vi "Bulk Delete Prompt.vi"(8 "error in (no error)":errorcluster, 11 "Item Ref in":T1 format="%.0x") -> (0 "error out":errorcluster)   [LabVIEW 2015, in "Modbus Master System Explorer.lvlib"]
uses:
  Modbus Master System Explorer.lvlib
  <vilib>/NI Veristand/Custom Device API/Custom Device Item Ref.ctl
  <vilib>/NI VeriStand/Custom Device API/Custom Device API.lvlib
panel:
  in  "Cancel":bool
  in  "Delete Selected":bool
  in  "Channels":i32[](listbox)
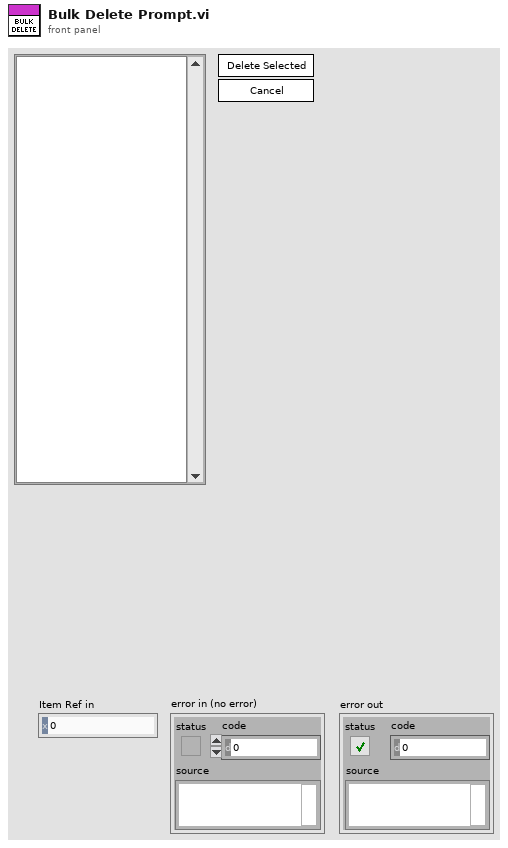
[diagram p1: front panel]
types:
  T1 = typedef "Custom Device API.lvlib/Custom Device Item Ref.ctl" = u64
  T2 = enum32{"Invalid", "Standard", "Closed", "Hidden", "Minimized", "Maximized"}
  T3 = typedef "Custom Device API.lvlib/Custom Device Item Info.ctl" = cluster{"Name":string, "Is Channel":bool, "GUID":string, "Is Waveform":bool}
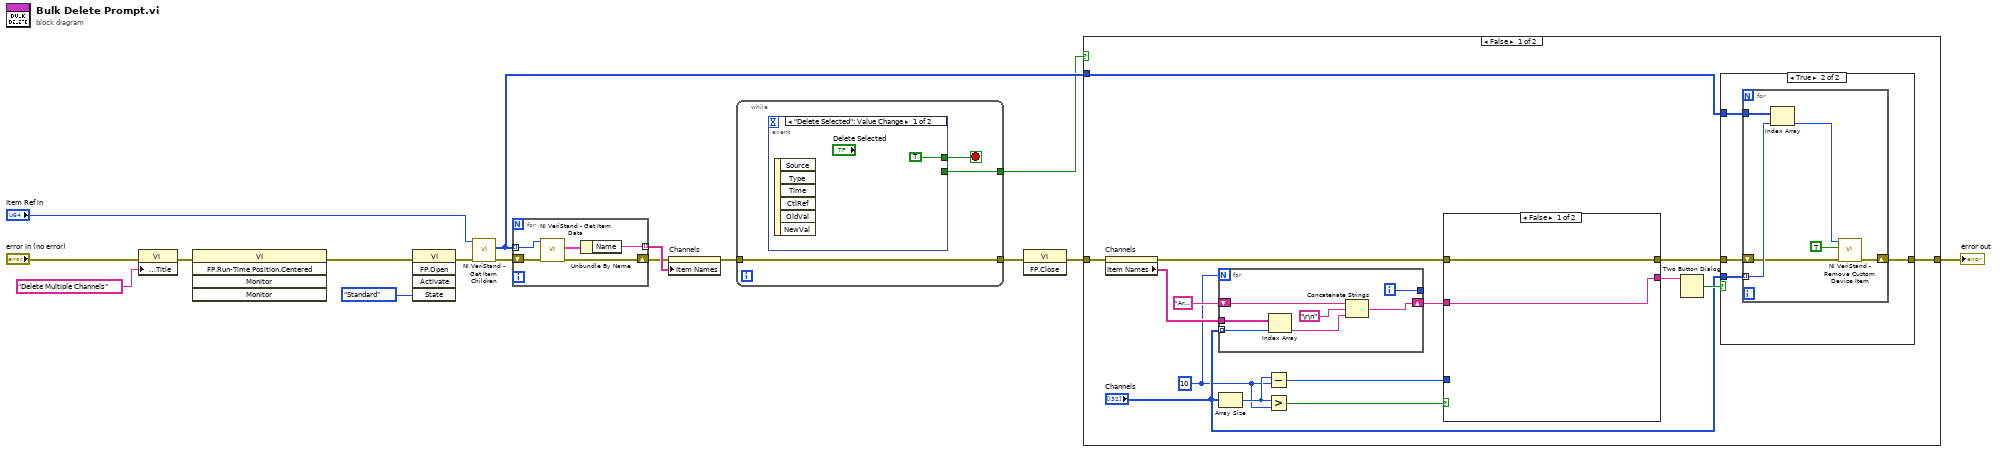
[diagram p0: block diagram]
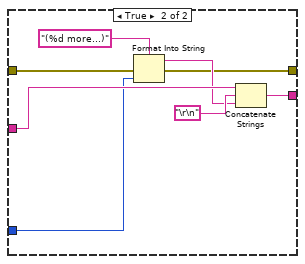
[diagram p2: hidden frame]
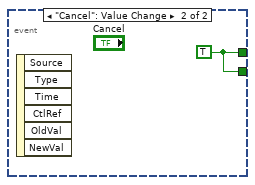
[diagram p5: hidden frame]
diagram:
  n1 = property class="VI"(error in="error in (no error)", "Front Panel.Title"="Delete Multiple Channels" ("Front Panel Window:Title")) -> (error out=w5:errorcluster)  [unwired: 1 in, 1 out]
  n2 = invoke class="VI" method="FP.Run-Time Position.Centered"(error in=w5) -> (error out=w4:errorcluster)  [unwired: 4 in, 4 out]
  n3 = invoke class="VI" method="FP.Open"(error in=w4, "State"=T2."Standard") -> (error out=w7:errorcluster)  [unwired: 3 in, 4 out]
  n4 = call <vilib>:"NI VeriStand - Get Item Children.vi"("error in (no error)"=w7, "Item Ref in"="Item Ref in") -> ("error out"=w15:errorcluster, "Child Refs"=w11:T1[])  [unwired: 6 in, 2 out]
  n5 = for {
    tunnel: w11 -> [w21] mode=indexing
    tunnel: [w19] -> w16 mode=indexing
    shift-right: [w17] -> w13
    shift-left: w15 -> [w18]
    n6 = call <vilib>:"NI VeriStand - Get Item Data.vi"("error in (no error)"=w18, "Item Ref in"=w21) -> ("error out"=w17:errorcluster, "Item Info"=w20:T3)  [unwired: 6 in, 2 out]
    n7 = Unbundle By Name(w20) -> ("Name"=w19:string)
  }
  n8 = property on="Channels" class="LstBox (strict)"(error in=w13, "Item Names"=w16) -> (error out=w12:errorcluster)  [unwired: 1 in, 1 out]
  n9 = while {
    tunnel: [w23] -> w10
    tunnel: w12 -> [w22]
    tunnel: [w22] -> w3
    stop <- w24 stop-if-true
    n10 = event shown="[0] \"Delete Selected\": Value Change" {
      selector: _ -> [_ _]
      dyn-events: _ -> [_ _]
      timeout: _ -> [_ _]
      tunnel: [TRUE w26] -> w24
      tunnel: [_ w26] -> w23
      event "Delete Selected": Value Change {
        n11 = event-data() -> ()  [unwired: 1 in, 6 out]
      }
      event "Cancel": Value Change {
        w26 = TRUE
        n12 = event-data() -> ()  [unwired: 1 in, 6 out]
      }
    }
  }
  n13 = invoke class="VI" method="FP.Close"(error in=w3) -> (error out=w2:errorcluster)  [unwired: 2 in, 2 out]
  n14 = case shown="False" w10 {
    tunnel: w11 -> [w41 _]
    tunnel: w2 -> [w29 w70]
    tunnel: [w40 w70] -> w1
    frame False {
      w30 = 10 ("x")
      n15 = property on="Channels" class="LstBox (strict)"(error in=w29) -> (error out=w28:errorcluster, "Item Names"=w39:string[])  [unwired: 1 in, 1 out]
      n16 = for {
        N: w30 -> [_]
        tunnel: w39 -> [w68]
        tunnel: "Channels" -> [w69] mode=indexing
        shift-right: [w65] -> w36
        shift-left: "Are you sure you want to delete the following channels?" -> [w67]
        tunnel: [w63] -> _
        i -> [w63]
        n17 = Index Array(array=w68, index=w69) -> (element=w64:string)
        n18 = Concatenate Strings(w67, "\r\n", w64) -> (w65:string)
      }
      n19 = Array Size(array="Channels") -> (size(s)=w32:i32)
      n20 = Subtract(x=w32, y=w30) -> (x-y=w35:i32)
      n21 = Greater?(x=w32, y=w30) -> (0:w31:bool)
      n22 = case shown="False" w31 {
        tunnel: w36 -> [w43 w51]
        tunnel: w35 -> [_ w48]
        tunnel: [w43 w46] -> w34
        tunnel: w28 -> [w42 w45]
        tunnel: [w42 w44] -> w27
        frame False {
        }
        frame True {
          n23 = Format Into String(format string="(%d more...)", error in=w45, w48) -> (resulting string=w47:string, error out=w44:errorcluster)  [unwired: 1 in]
          n24 = Concatenate Strings(w51, "\r\n", w47) -> (w46:string)
        }
      }
      n25 = Two Button Dialog(message=w34) -> (T button?=w37:bool)  [unwired: 2 in]
      n26 = case shown="True" w37 {
        tunnel: w41 -> [_ w56]
        tunnel: w27 -> [w52 w55]
        tunnel: [w52 w54] -> w40
        tunnel: "Channels" -> [_ w53]
        frame False {
        }
        frame True {
          n27 = for {
            tunnel: w53 -> [w61] mode=indexing
            tunnel: w56 -> [w62]
            shift-right: [w57] -> w54
            shift-left: w55 -> [w58]
            n28 = Index Array(array=w62, index=w61) -> (element=w60:T1)
            n29 = call <vilib>:"NI VeriStand - Remove Custom Device Item.vi"("error in (no error)"=w58, "Force Delete (F)"=TRUE, "Item Ref in"=w60) -> ("error out"=w57:errorcluster)  [unwired: 7 in, 1 out]
          }
        }
      }
    }
    frame True {
    }
  }
  "error out" <- w1
